vi "Handle Controller.vi"(7 "Processing In":refnum<class "Processing.lvclass">, 10 "Controller in":refnum<class "Controller.lvclass">, 11 "Arguments Handler in":refnum<class "Controller Handler.lvclass">) -> (0 "error out":errorcluster, 2 "Controller":refnum<class "Controller.lvclass">, 5 "Processing":refnum<class "Processing.lvclass">)   [LabVIEW 2020, in "HTTP Server.lvlib" / "Controller Handler.lvclass"]
uses:
  Controller Handler.lvclass
  Processing/Processing.lvclass
  Controller/Controller.lvclass
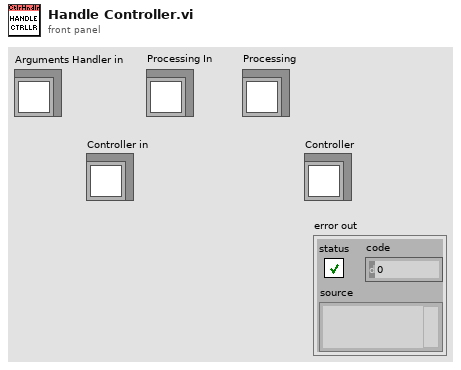
[diagram p1: front panel]
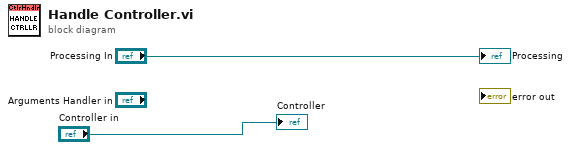
[diagram p0: block diagram]
diagram:
  "Processing" <- "Processing In"
  "Controller" <- "Controller in"
